vi "Image Generator.vi"(9 "Assembly Line Input":refnum<class "Assembly Line Input.lvclass">, 10 "how many":i32=50, 11 "Queue in":refnum<queue>) -> (0 "error out":errorcluster)   [LabVIEW 2018, in "Assembly Line Input.lvclass"]
doc: "Given an image for a correct board, generate the requested number of randomly correct or incorrect image (with approximately 75% success rate) and add them to the queue."
uses:
  Classes/Assembly Line Input_class/Assembly Line Input.lvclass
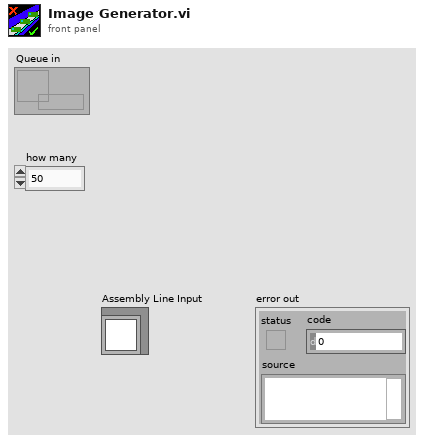
[diagram p1: front panel]
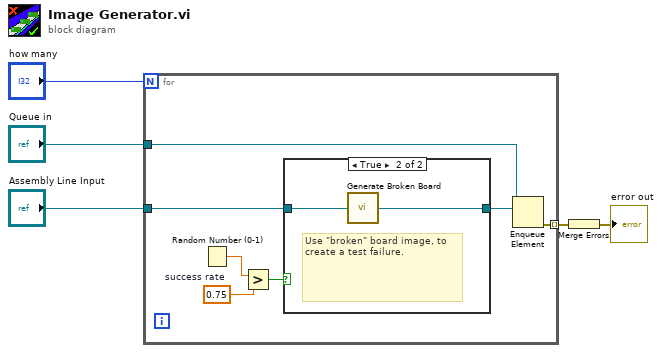
[diagram p0: block diagram]
diagram:
  n1 = for {
    N: "how many" -> [_]
    tunnel: "Queue in" -> [w12]
    tunnel: "Assembly Line Input" -> [w8]
    tunnel: [w6] -> w2 mode=indexing
    w10 = 0.75  # success rate
    n2 = Random Number (0-1)() -> (number: 0 to 1=w11:dbl)
    n3 = Greater?(x=w11, y=w10) -> (0:w9:bool)
    n4 = case shown="True" w9 {
      tunnel: w8 -> [w13 w15]
      tunnel: [w13 w14] -> w7
      frame False {
        # "Use \"correct\" image from input."
      }
      frame True {
        # "Use \"broken\" board image, to create a test failure."
        n5 = call "Generate Broken Board.vi"("Assembly Line Input in"=w15) -> ("Assembly Line Input out"=w14:refnum<class "Assembly Line Input.lvclass">)
      }
    }
    n6 = Enqueue Element(queue=w12, element=w7) -> (error out=w6:errorcluster)  [unwired: 2 in, 2 out]
  }
  n7 = Merge Errors(w2) -> (→"error out":errorcluster)
